vi "about process module notes.vi"(8 "error in (no error)":errorcluster, 11 "Notes Path (empty)":path) -> (0 "error out":errorcluster, 3 "release notes obj":string)   [LabVIEW 2011]
uses:
  <vilib>/Utility/config.llb/NI_LVConfig.lvlib
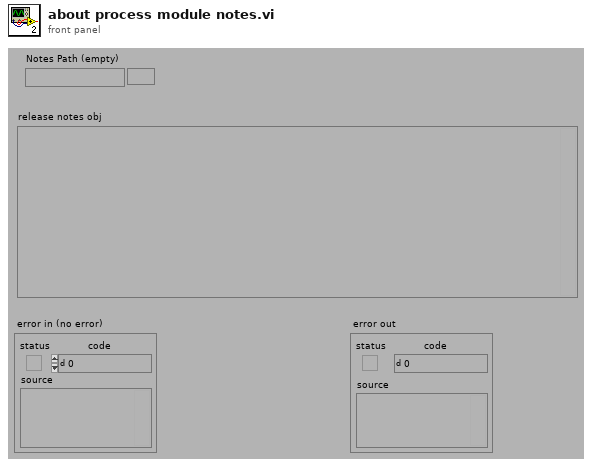
[diagram p1: front panel]
types:
  T1 = typedef "NI_LVConfig.lvlib/Config Data RefNum.ctl" = refnum<k1>
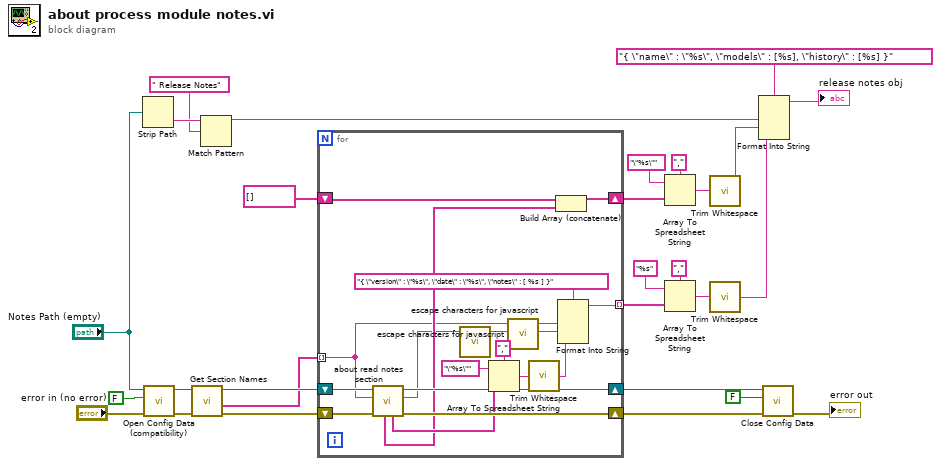
[diagram p0: block diagram]
diagram:
  n1 = Strip Path(path="Notes Path (empty)") -> (name=w9:string)  [unwired: 1 out]
  n2 = call <vilib>:"Open Config Data (compatibility).vi"("error in (no error)"="error in (no error)", "create file if necessary (T)"=FALSE, "configuration file path"="Notes Path (empty)") -> ("error out"=w25:errorcluster, "refnum"=w26:T1)  [unwired: 6 in, 1 out]
  n3 = call <vilib>:"Get Section Names.vi"("error in (no error)"=w25, "refnum"=w26) -> ("error out"=w18:errorcluster, "section names"=w16:string[], "refnum out"=w19:T1)  [unwired: 7 out]
  n4 = Match Pattern(string=w9, regular expression=" Release Notes") -> (before substring=w8:string)  [unwired: 4 out]
  n5 = for {
    shift-right: [w44] -> w23
    shift-left: w18 -> [w45]
    tunnel: w16 -> [w32] mode=indexing
    shift-right: [w43] -> w24
    shift-left: w19 -> [w46]
    tunnel: [w36] -> w14 mode=indexing
    shift-right: [w34] -> w2
    shift-left: string[] [] -> [w35]
    n6 = call "about read notes section.vi"("error in (no error)"=w45, "Section Name (\"\")"=w32, "refnum"=w46) -> ("error out"=w44:errorcluster, "Date"=w30:string, "dup refnum"=w43:T1, "Notes"=w38:string[], "Models"=w33:string[])  [unwired: 1 in, 3 out]
    n7 = call "escape characters for javascript.vi"("String (\"\")"=w30) -> ("escaped String"=w29:string)  [unwired: 4 out]
    n8 = Array To Spreadsheet String(delimiter (Tab)=",", array=w38, 3:"\"%s\"" ("format string")) -> (spreadsheet string=w39:string)
    n9 = call "escape characters for javascript.vi"("String (\"\")"=w32) -> ("escaped String"=w31:string)  [unwired: 4 out]
    n10 = call <vilib>:"Trim Whitespace.vi"("string"=w39) -> ("trimmed string"=w37:string)  [unwired: 1 in]
    n11 = Build Array (concatenate)(w35, w33) -> (w34:string[])
    n12 = Format Into String(format string="{ \"version\" : \"%s\", \"date\" : \"%s\", \"notes\" : [ %s ] }", w31, w29, w37) -> (resulting string=w36:string)  [unwired: 2 in, 1 out]
  }
  n13 = Array To Spreadsheet String(delimiter (Tab)=",", array=w2, 3:"\"%s\"") -> (spreadsheet string=w4:string)
  n14 = Array To Spreadsheet String(delimiter (Tab)=",", array=w14, 3:"%s") -> (spreadsheet string=w13:string)
  n15 = call <vilib>:"Trim Whitespace.vi"("string"=w4) -> ("trimmed string"=w1:string)  [unwired: 1 in]
  n16 = call <vilib>:"Trim Whitespace.vi"("string"=w13) -> ("trimmed string"=w12:string)  [unwired: 1 in]
  n17 = Format Into String(format string="{ \"name\" : \"%s\", \"models\" : [%s], \"history\" : [%s] }", w8, w1, w12) -> (resulting string=→"release notes obj":string)  [unwired: 2 in, 1 out]
  n18 = call <vilib>:"Close Config Data.vi"("error in (no error)"=w23, "write file if changed (T)"=FALSE, "refnum"=w24) -> ("error out"=→"error out":errorcluster)  [unwired: 8 out]
